vi "SimulationData.vi"() -> ()   [LabVIEW 2009, in "Host.lvlib"]
uses:
  Host.lvlib
  <vilib>/Platform/TimedLoop/XDataNode/XDataNode.xnode
  <vilib>/Platform/TimedLoop/XDataNode/loadlvalarms.vi
  <vilib>/Platform/TimedLoop/XDataNode/timing_clust.ctl
  <vilib>/Platform/TimedLoop/XDataNode/nitl_modes.ctl
  <vilib>/Platform/TimedLoop/XDataNode/wakeup.ctl
  <vilib>/Platform/TimedLoop/XDataNode/XDNodeRunTimeDep.lvlib
panel:
  in  "stop":bool
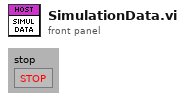
[diagram p1: front panel]
types:
  T1 = cluster{"Position":cluster{"X":dbl, "Y":dbl, "Angle":dbl}, "Speed":cluster{"Left":dbl, "Right":dbl}}
  T2 = typedef "XDNodeRunTimeDep.lvlib/timing_clust.ctl" = cluster{"Expected End [f-1]":u64, "Actual End [f-1]":u64, "Finished Late? [f-1]":bool, "Expected End [i-1]":u64, "Actual End [i-1]":u64, "Finished Late? [i-1]":bool, "Expected Start [i]":u64, "Actual Start [i]":u64, "Expected Start [f]":u64, "Actual Start [f]":u64, "Source Name":string, "Structure Name":string, "Period":i64, "Deadline":i64, "Offset":i64, "Start":i64, "Priority":i32, "Timeout":i32, "Mode":T3, "Wakeup Reason":T4, "Error":errorcluster, "Source Type":string, "Secondary Source Type":string, "Global End Time":u64, "Global Start Time":u64, "Frame Duration":u64, "Iteration Duration":u64, "Assigned CPU":i32, "I/O Scan Engine Mode":u32}
  T3 = typedef "XDNodeRunTimeDep.lvlib/nitl_modes.ctl" = enum32{"No Change", "Process missed periods, maintain original phase", "Discard missed periods, maintain original phase", "Process missed periods, ignore original phase", "Discard missed periods, ignore original phase"}
  T4 = typedef "XDNodeRunTimeDep.lvlib/wakeup.ctl" = enum32{"Normal", "Aborted", "Asynchronous wakeup", "Timing source error", "Timed loop error", "Timeout"}
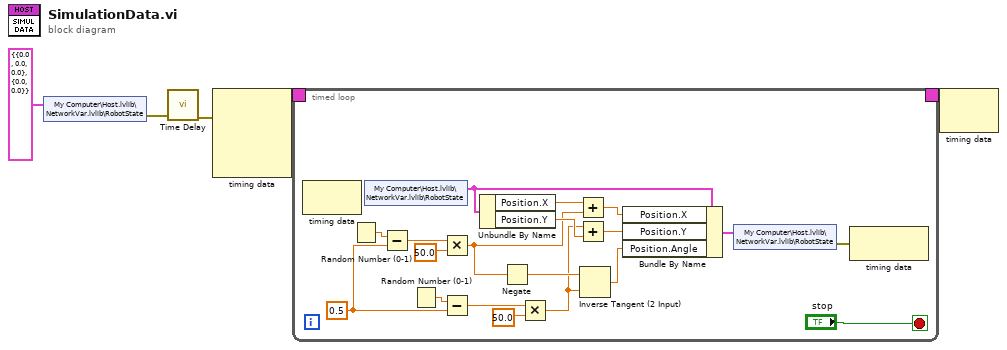
[diagram p0: block diagram]
diagram:
  n1 = shared-variable "My Computer\\Host.lvlib\\NetworkVar.lvlib\\RobotState"(T1 {"Position"={"X"=0.0, "Y"=0.0, "Angle"=0.0}, "Speed"={"Left"=0.0, "Right"=0.0}} ("RobotState")) -> (error out=w2:errorcluster)  [unwired: 1 in]
  n2 = call "Time Delay"("error in (no error)"=w2) -> ("error out"=w1:errorcluster)  [unwired: 10 in]
  n3 = node-c288(w1) -> (w5:T2)  [unwired: 3 in]
  n4 = timed-loop {
    timing: w5 -> [_]
    timing-out: [_] -> w4
    stop <- "stop" stop-if-true
    w13 = 0.5 ("y")
    n5 = node-c288() -> ()  [unwired: 1 in, 1 out]
    n6 = Random Number (0-1)() -> (number: 0 to 1=w14:dbl)
    n7 = shared-variable "My Computer\\Host.lvlib\\NetworkVar.lvlib\\RobotState"() -> (w10:T1)  [unwired: 1 in, 1 out]
    n8 = Subtract(x=w14, y=w13) -> (x-y=w16:dbl)
    n9 = Random Number (0-1)() -> (number: 0 to 1=w20:dbl)
    n10 = Multiply(x=w16, y=50.0) -> (x*y=w7:dbl)
    n11 = Subtract(x=w20, y=w13) -> (x-y=w18:dbl)
    n12 = Unbundle By Name(w10) -> ("Position.X"=w12:dbl, "Position.Y"=w22:dbl)
    n13 = Negate(x=w7) -> (-x=w8:dbl)
    n14 = Multiply(x=w18, y=50.0) -> (x*y=w6:dbl)
    n15 = Add(x=w12, y=w7) -> (x+y=w11:dbl)
    n16 = Add(x=w6, y=w22) -> (x+y=w19:dbl)
    n17 = Inverse Tangent (2 Input)(1:w6, 2:w8) -> (0:w9:dbl)
    n18 = Bundle By Name(cluster=w10, "Position.X"=w11, "Position.Y"=w19, "Position.Angle"=w9) -> (w24:T1)
    n19 = shared-variable "My Computer\\Host.lvlib\\NetworkVar.lvlib\\RobotState"(w24) -> (error out=w23:errorcluster)  [unwired: 1 in]
    n20 = node-c288(w23) -> ()  [unwired: 1 out]
  }
  n21 = node-c288(w4) -> ()  [unwired: 1 out]
